vi "Get Camera Event Status.vi"(11 "camStatus":u32) -> (2 "function return":u32, 3 "camStatus out":u32)   [LabVIEW 2018, in "AndorSDK.lvlib"]
doc: "EXPNETTYPE unsigned int WINAPI GetCameraEventStatus(DWORD * camStatus);"
uses:
  AndorSDK.lvlib
  ATMCD32D.dll
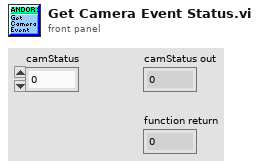
[diagram p1: front panel]
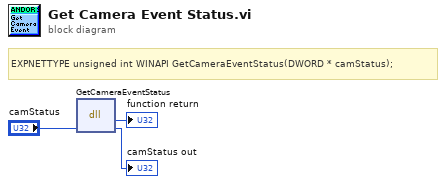
[diagram p0: block diagram]
diagram:
  # "EXPNETTYPE unsigned int WINAPI GetCameraEventStatus(DWORD * camStatus);"
  n1 = dll-call lib="PTH2babs E\nPersönliches02 - Arbeit03-HiwijobsLabviewCodelibANDOR\tAndor SDK\nATMCD32D.*" fn="GetCameraEventStatus"("camStatus"="camStatus") -> (→"function return":u32, "camStatus"=→"camStatus out":u32)  [unwired: 3 in, 2 out]
